vi "稳定T？.vi"(7 "次数(100)":dbl=100.0 format="%#_13g", 10 "Reset":bool, 11 "输入":bool) -> (3 "TT？":bool)   [LabVIEW 2017]
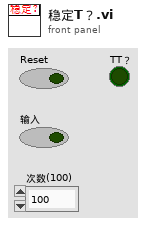
[diagram p1: front panel]
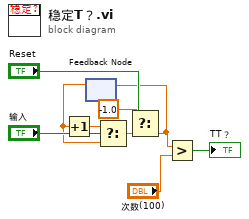
[diagram p0: block diagram]
diagram:
  n1 = feedback #1() -> (w2:dbl)  [unwired: 1 in]
  n2 = Increment(x=w2) -> (x+1=w1:dbl)
  n3 = Select(t=w1, s="输入", f=w2) -> (s? t:f=w3:dbl)
  n4 = Select(t=-1.0, s="Reset", f=w3) -> (s? t:f=w7:dbl)
  n5 = feedback-in #1(w7) -> ()
  n6 = Greater?(x=w7, y="次数(100)") -> (0:→"TT？":bool)
